vi "Begin.vi"() -> (0 "error out":errorcluster)   [LabVIEW 2013]
doc: "Called before other user functions, this VI is expected to open initial I/O refnums, load in file data, and do all program initialization. Notice that the <B>error out</B> terminal is simply used for data flow. Wiring it to other structures or subVIs ensures that this VI runs first."
uses:
  <vilib>/Rock Robotics/WPI/DriverStation/WPI_DriverStationRobotMode2.ctl
  <vilib>/Rock Robotics/WPI/Joystick/WPI_JoystickDeviceEnum.ctl
  <vilib>/Rock Robotics/SystemInterfaces/DIO/FPGA_DIOChannel.ctl
  <vilib>/Rock Robotics/SystemInterfaces/DIO/FPGA_DIORelayChannel.ctl
  <vilib>/Rock Robotics/SystemInterfaces/AI/FPGA_AIChannel.ctl
  <vilib>/Rock Robotics/SystemInterfaces/AI/FPGA_AIGyroChannel.ctl
  <vilib>/Rock Robotics/SystemInterfaces/Typedef/FPGA_TypedefAnalogModuleForGyro.ctl
  <vilib>/Rock Robotics/SystemInterfaces/Typedef/FPGA_TypedefDigitalModule.ctl
  <vilib>/Rock Robotics/SystemInterfaces/DIO/FPGA_DIOPWMChannel.ctl
  <vilib>/Rock Robotics/WPI/SafetyOutput/WPI_SafetyOutputConfigMenu.ctl
  <vilib>/Rock Robotics/WPI/Solenoid/WPI_SolenoidChannel.ctl
  <vilib>/Rock Robotics/WPI/Relay/WPI_RelayValue.ctl
  <vilib>/Rock Robotics/SystemInterfaces/Typedef/FPGA_TypedefAnalogModule.ctl
  <vilib>/Rock Robotics/WPI/Solenoid/WPI_SolenoidValue.ctl
  Robot Global Data.vi
  <vilib>/Rock Robotics/WPI/Counter/WPI_CounterDigitalInputToDigitalSource.vi
  <vilib>/Rock Robotics/WPI/RobotDrive/WPI_RobotDriveOpen2MotorWithTalon.vi
  <vilib>/Rock Robotics/WPI/MotorControl/WPI_MotorControlOpen Talon.vi
  <vilib>/Rock Robotics/WPI/Solenoid/WPI_SolenoidOpenSingle.vi
  <vilib>/Rock Robotics/WPI/Solenoid/WPI_SolenoidSetEnum.vi
  <vilib>/Rock Robotics/WPI/Compressor/WPI_CompressorGetSetRefNum.vi
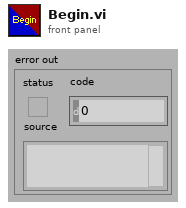
[diagram p1: front panel]
types:
  T1 = typedef "FPGA_DIOChannel.ctl" = enum8{"DIO 1", "DIO 2", "DIO 3", "DIO 4", "DIO 5", "DIO 6", "DIO 7", "DIO 8", "DIO 9", "DIO 10", "DIO 11", "DIO 12", "DIO 13", "DIO 14", "Invalid"}
  T2 = typedef "WPI_SolenoidChannel.ctl" = enum8{"Solenoid 1", "Solenoid 2", "Solenoid 3", "Solenoid 4", "Solenoid 5", "Solenoid 6", "Solenoid 7", "Solenoid 8", "Invalid"}
  T3 = typedef "WPI_SolenoidValue.ctl" = enum16{"Off", "On", "Forward", "Reverse"}
  T4 = typedef "FPGA_TypedefAnalogModule.ctl" = enum16{"Analog Module 1", "Analog Module 2"}
  T5 = typedef "FPGA_DIORelayChannel.ctl" = enum8{"Relay 1", "Relay 2", "Relay 3", "Relay 4", "Relay 5", "Relay 6", "Relay 7", "Relay 8", "Invalid"}
  T6 = typedef "WPI_RelayValue.ctl" = enum16{"Off", "On", "Forward", "Reverse"}
  T7 = typedef "FPGA_DIOPWMChannel.ctl" = enum8{"PWM 1", "PWM 2", "PWM 3", "PWM 4", "PWM 5", "PWM 6", "PWM 7", "PWM 8", "PWM 9", "PWM 10", "Invalid"}
  T8 = typedef "WPI_SafetyOutputConfigMenu.ctl" = enum16{"Enable", "Disable"}
  T9 = typedef "FPGA_TypedefDigitalModule.ctl" = enum16{"Digital Module 1", "Digital Module 2"}
  T10 = typedef "FPGA_TypedefAnalogModuleForGyro.ctl" = enum16{"Analog Module 1"}
  T11 = typedef "FPGA_AIGyroChannel.ctl" = enum8{"AI 1", "AI 2", "Invalid"}
  T12 = typedef "FPGA_AIChannel.ctl" = enum8{"AI 1", "AI 2", "AI 3", "AI 4", "AI 5", "AI 6", "AI 7", "AI 8", "Invalid"}
  T13 = typedef "WPI_JoystickDeviceEnum.ctl" = enum16{"USB 1", "USB 2", "USB 3", "USB 4", "Kinect 1", "Kinect 2"}
  T14 = typedef "WPI_DriverStationRobotMode2.ctl" = enum16{"Autonomous Disabled", "Autonomous Enabled", "Teleop Disabled", "Teleop Enabled", "Timeout", "Finish", "Test Disabled", "Test Enabled"}
  T15 = typedef "WPI_JoystickDevRef.ctl" = cluster{"Device":T13}
  T16 = typedef "WPI_SolenoidDevRef.ctl" = cluster{"DevStatus":errorcluster, "Solenoid Module":T17, "Forward Solenoid Channel":T2, "Reverse Solenoid Channel":T2}
  T17 = typedef "FPGA_TypedefSolenoidModule.ctl" = enum16{"Solenoid Module 1", "Solenoid Module 2"}
  T18 = typedef "WPI_CompressorDevRef.ctl" = cluster{"DevStatus":errorcluster, "DigitalInputDevRef":T19, "RelayDevRef":T20}
  T19 = typedef "WPI_DigitalInputDevRef.ctl" = cluster{"DevStatus":errorcluster, "DIO Channel":T1, "Digital Module":T9}
  T20 = typedef "WPI_RelayDevRef.ctl" = cluster{"DevStatus":errorcluster, "Relay Channel":T5, "Digital Module":T9, "Relay Direction":T21}
  T21 = typedef "WPI_RelayDirection.ctl" = enum16{"Both directions", "Forward only", "Reverse only"}
  T22 = typedef "FPGA_CounterEncoderSourceConvertionLVSourceType.ctl" = cluster{"DevStatus":errorcluster, "AnalogTriggerMode?":bool, "DigitalMode":cluster{"Digital Module":T9, "DIO Channel":T23}, "AnalogTriggerMode":cluster{"AnalogTriggerIndex":T24, "OutputType":T25}}
  T23 = typedef "FPGA_DIODigitalSourceChannel.ctl" = enum8{"DIO 1", "DIO 2", "DIO 3", "DIO 4", "DIO 5", "DIO 6", "DIO 7", "DIO 8", "DIO 9", "DIO 10", "DIO 11", "DIO 12", "DIO 13", "DIO 14", "Disabled"}
  T24 = typedef "FPGA_AnalogTriggerIndex.ctl" = enum8{"Trig 0", "Trig 1", "Trig 2", "Trig 3", "Trig 4", "Trig 5", "Trig 6", "Trig 7", "Invalid"}
  T25 = typedef "FPGA_AnalogTriggerOutType.ctl" = enum16{"InWindow", "TriggerState", "Rising", "Falling"}
  T26 = typedef "WPI_MotorControlDeviceRef.ctl" = cluster{"DeviceStatus":errorcluster, "Type":enum16{"PWM", "CAN"}, "PWM":cluster{"Digital Module":T9, "PWM Channel":T7, "DeadBand":T27}, "CAN":cluster{"Device Number":u8, "Control Mode":T28, "Semaphore":T29, "Max Vout":dbl}, "Invert":bool, "TransformRef":T30, "InvTransformRef":T30}
  T27 = typedef "WPI_PWMDeadband.ctl" = cluster{"Name":string, "maxPositivePwm":i32, "minPositivePwm":i32, "centerPwm":i32, "maxNegativePwm":i32, "minNegativePwm":i32, "angularRange":u16}
  T28 = typedef "WPI_CANJaguar_ControlMode.ctl" = enum8{"Percent VBus", "Current", "Speed", "Position", "Voltage"}
  T29 = typedef "Semaphore RefNum" = refnum<k1>
  T30 = typedef "WPI_PWMTransform_ConPane.ctl" = refnum<vi>
  T31 = typedef "WPI_RobotDriveDevRef.ctl" = cluster{"DevStatus":errorcluster, "Motors[]":T26[], "Square Inputs":bool, "Max Output":dbl, "Isochronous":bool}
  T32 = typedef "WPI_EncoderDevRef.ctl" = cluster{"DevStatus":errorcluster, "EncoderIndex":T33, "CounterIndex":T34, "DistancePerCount":dbl, "Decoding Type":T35}
  T33 = typedef "FPGA_EncoderIdx.ctl" = enum8{"Enc 0", "Enc 1", "Enc 2", "Enc 3", "Invalid"}
  T34 = typedef "FPGA_CounterCtrSystemIndex.ctl" = enum8{"Ctr 0", "Ctr 1", "Ctr 2", "Ctr 3", "Ctr 4", "Ctr 5", "Ctr 6", "Ctr 7", "Invalid"}
  T35 = typedef "WPI_EncoderType.ctl" = enum16{"1x", "2x", "4x"}
  T36 = typedef "WPI_AnalogChannelDevRef.ctl" = cluster{"DevStatus":errorcluster, "Analog Module":T4, "Analog Channel":T12}
  T37 = typedef "WPI_GyroDevRef.ctl" = cluster{"DevStatus":errorcluster, "Analog Module":T4, "Analog Channel":T12, "Offset":dbl, "Gain (VoltsPerDegree/Second)":dbl}
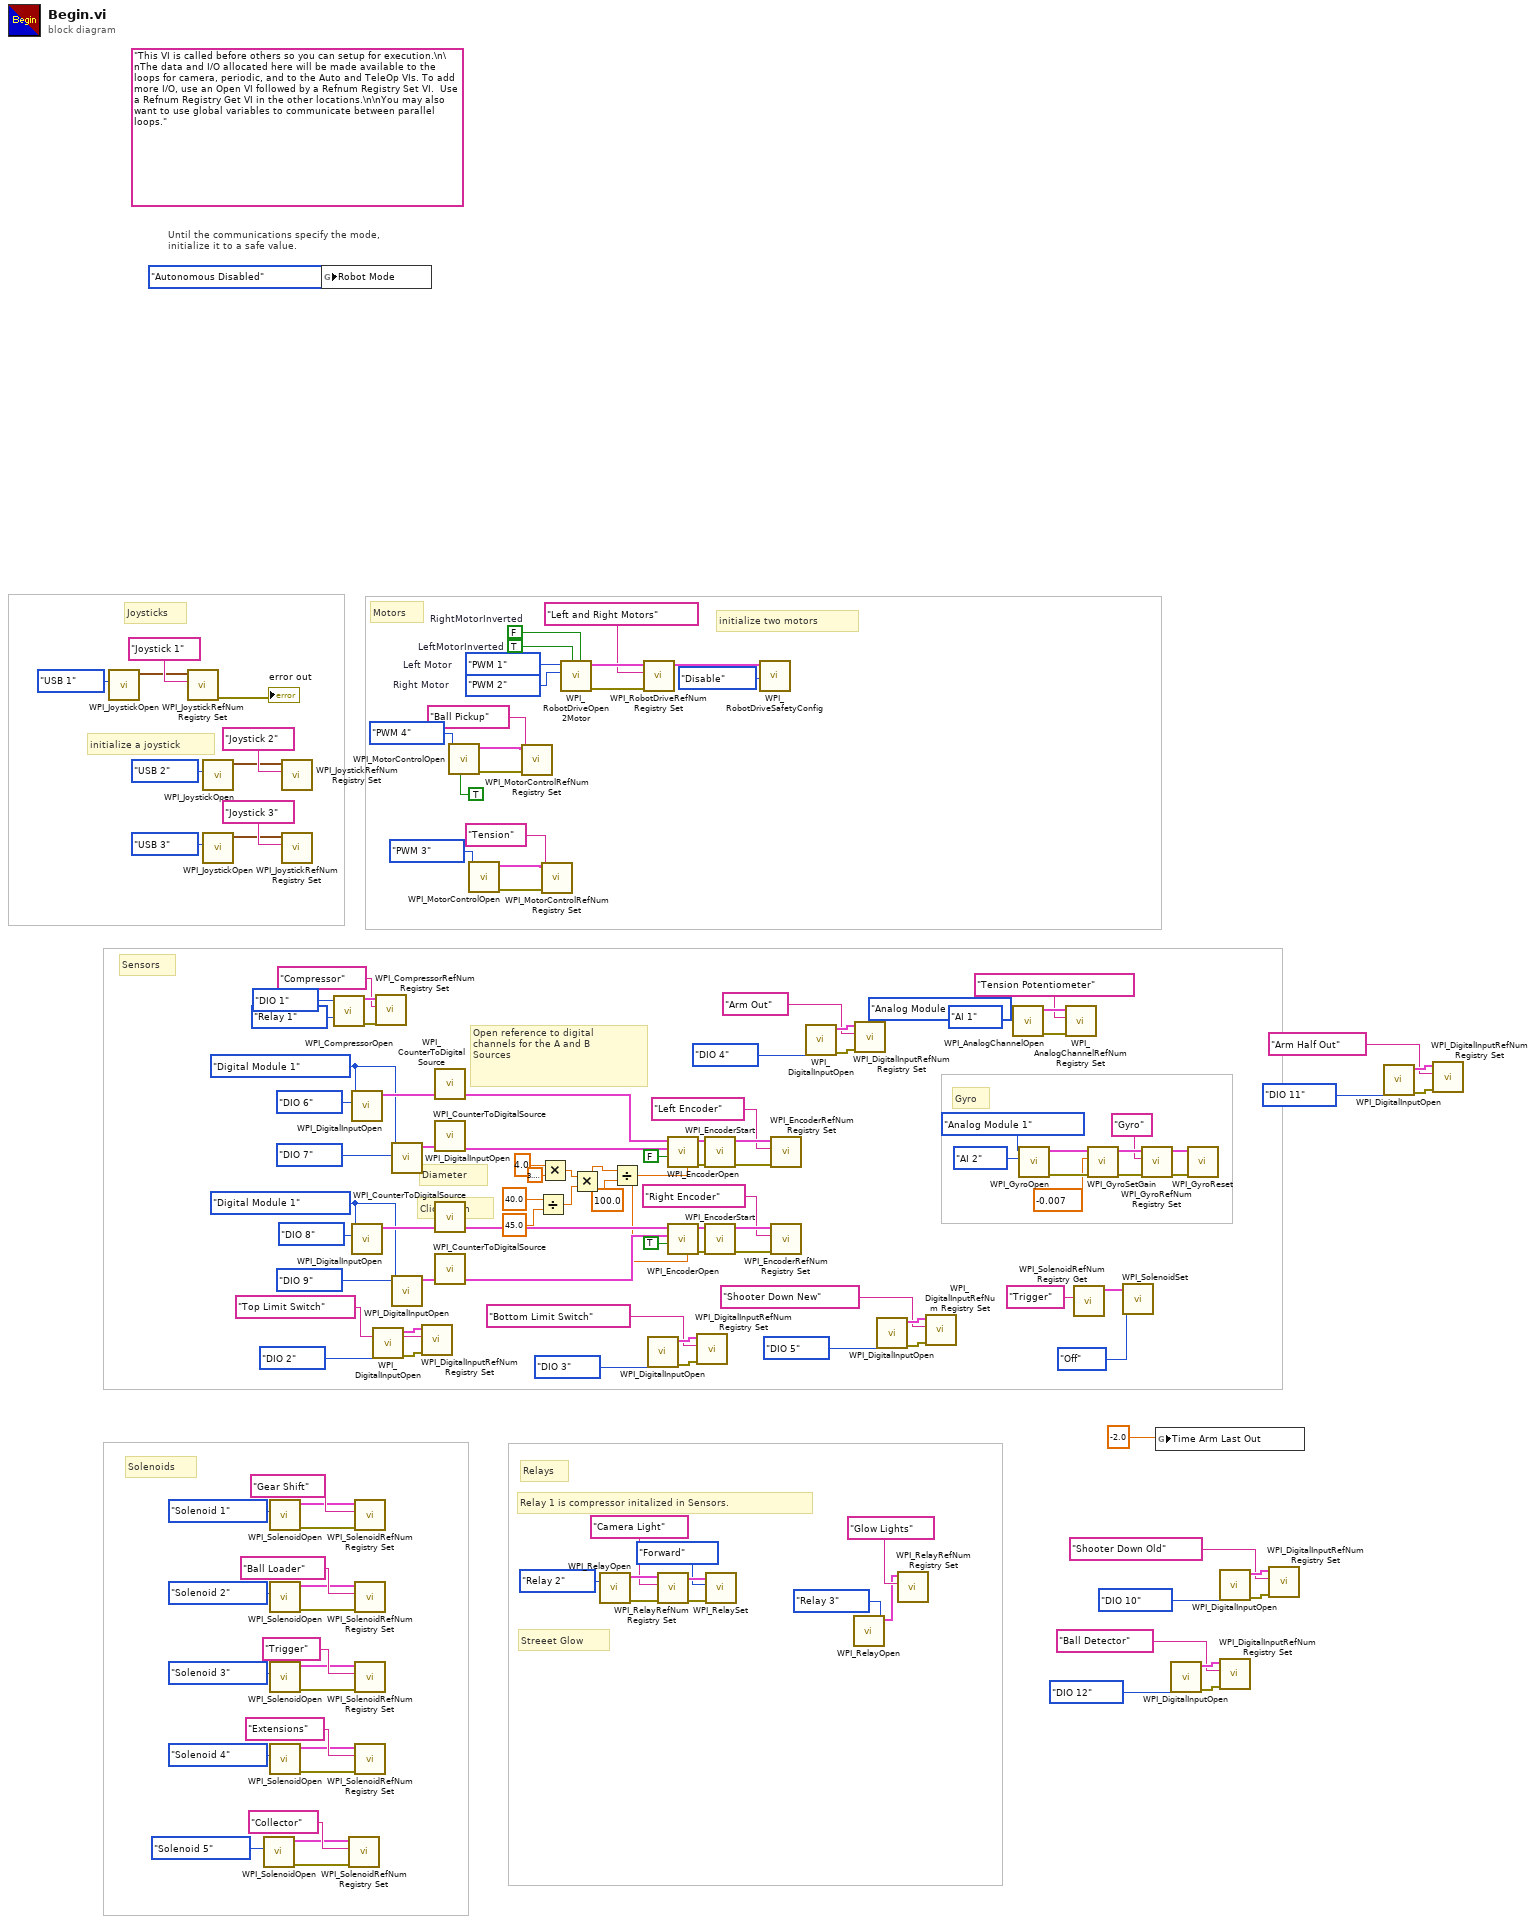
[diagram p0: block diagram]
diagram:
  w82 = FPGA_DIOPWMChannel."PWM 2"  # Right Motor
  w83 = FPGA_DIOPWMChannel."PWM 1"  # Left Motor
  w87 = TRUE  # LeftMotorInverted
  w88 = FALSE  # RightMotorInverted
  w96 = FPGA_TypedefDigitalModule."Digital Module 1" ("DIO Module 2")
  w103 = FPGA_TypedefDigitalModule."Digital Module 1" ("DIO Module")
  (unwired) "This VI is called before others so you can setup for execution.\n\nThe data and I/O allocated here will be made available to the loops for camera, periodic, and to the Auto and TeleOp VIs. To add more I/O, use an Open VI followed by a Refnum Registry Set VI.  Use a Refnum Registry Get VI in the other locations.\n\nYou may also want to use global variables to communicate between parallel loops."
  # "Streeet Glow"
  # "Relay 1 is compressor initalized in Sensors."
  # "Relays"
  # "Solenoids"
  # "Motors"
  # "initialize two motors"
  # "Clicks/inch"
  # "Diameter"
  # "Open reference to digital \nchannels for the A and B\nSources"
  # "Gyro"
  # "Sensors"
  # "Joysticks"
  # "initialize a joystick"
  # "Until the communications specify the mode,\ninitialize it to a safe value."
  n1 = call <vilib>:"WPI_JoystickOpen.vi"("JoystickDevice"=WPI_JoystickDeviceEnum."USB 1") -> ("JoystickDevRef"=w144:T15)  [unwired: 10 in]
  n2 = call <vilib>:"WPI_JoystickRefNum Registry Set.vi"("refnum name"="Joystick 1", "JoystickDevRef"=w144) -> ("error out"=→"error out":errorcluster)  [unwired: 8 in, 1 out]
  n3 = call <vilib>:"WPI_JoystickOpen.vi"("JoystickDevice"=WPI_JoystickDeviceEnum."USB 2") -> ("JoystickDevRef"=w140:T15)  [unwired: 10 in]
  n4 = call <vilib>:"WPI_JoystickOpen.vi"("JoystickDevice"=WPI_JoystickDeviceEnum."USB 3") -> ("JoystickDevRef"=w137:T15)  [unwired: 10 in]
  n5 = call-poly <vilib>:"WPI_SolenoidOpen.vi"("Solenoid Channel"=WPI_SolenoidChannel."Solenoid 5") -> ("error out"=w19:errorcluster, "SolenoidDevRef"=w20:T16)  [unwired: 9 in]
  n6 = call-poly <vilib>:"WPI_SolenoidOpen.vi"("Solenoid Channel"=WPI_SolenoidChannel."Solenoid 1") -> ("error out"=w55:errorcluster, "SolenoidDevRef"=w56:T16)  [unwired: 9 in]
  n7 = call-poly <vilib>:"WPI_SolenoidOpen.vi"("Solenoid Channel"=WPI_SolenoidChannel."Solenoid 2") -> ("error out"=w59:errorcluster, "SolenoidDevRef"=w60:T16)  [unwired: 9 in]
  n8 = call-poly <vilib>:"WPI_SolenoidOpen.vi"("Solenoid Channel"=WPI_SolenoidChannel."Solenoid 3") -> ("error out"=w63:errorcluster, "SolenoidDevRef"=w64:T16)  [unwired: 9 in]
  n9 = call-poly <vilib>:"WPI_SolenoidOpen.vi"("Solenoid Channel"=WPI_SolenoidChannel."Solenoid 4") -> ("error out"=w67:errorcluster, "SolenoidDevRef"=w68:T16)  [unwired: 9 in]
  n10 = call <vilib>:"WPI_JoystickRefNum Registry Set.vi"("refnum name"="Joystick 2", "JoystickDevRef"=w140) -> ()  [unwired: 8 in, 2 out]
  n11 = call <vilib>:"WPI_JoystickRefNum Registry Set.vi"("refnum name"="Joystick 3", "JoystickDevRef"=w137) -> ()  [unwired: 8 in, 2 out]
  n12 = global write "Robot Global Data.vi" "Robot Mode"(WPI_DriverStationRobotMode2."Autonomous Disabled" ("Robot Mode")) -> ()
  n13 = call <vilib>:"WPI_CompressorOpen.vi"("Pressure Switch DIO Channel"=FPGA_DIOChannel."DIO 1", "Relay Channel"=FPGA_DIORelayChannel."Relay 1") -> ("CompressorDevRef"=w134:T18, "error out"=w135:errorcluster)  [unwired: 12 in]
  n14 = call <vilib>:"WPI_SolenoidRefNum Registry Set.vi"("error in (no error)"=w19, "refnum name"="Collector", "SolenoidDevRef"=w20) -> ()  [unwired: 7 in, 2 out]
  n15 = call <vilib>:"WPI_DigitalInputOpen.vi"("DIO Channel"=FPGA_DIOChannel."DIO 6" ("A Channel"), "Digital Module (Module 1)"=w103) -> ("DigitalInputDevRef"=w106:T19)  [unwired: 1 in, 8 out]
  n16 = call <vilib>:"WPI_DigitalInputOpen.vi"("DIO Channel"=FPGA_DIOChannel."DIO 8" ("A Channel 2"), "Digital Module (Module 1)"=w96) -> ("DigitalInputDevRef"=w99:T19)  [unwired: 1 in, 8 out]
  n17 = call <vilib>:"WPI_SolenoidRefNum Registry Set.vi"("error in (no error)"=w55, "refnum name"="Gear Shift", "SolenoidDevRef"=w56) -> ()  [unwired: 7 in, 2 out]
  n18 = call <vilib>:"WPI_SolenoidRefNum Registry Set.vi"("error in (no error)"=w59, "refnum name"="Ball Loader", "SolenoidDevRef"=w60) -> ()  [unwired: 7 in, 2 out]
  n19 = call <vilib>:"WPI_SolenoidRefNum Registry Set.vi"("error in (no error)"=w63, "refnum name"="Trigger", "SolenoidDevRef"=w64) -> ()  [unwired: 7 in, 2 out]
  n20 = call <vilib>:"WPI_SolenoidRefNum Registry Set.vi"("error in (no error)"=w67, "refnum name"="Extensions", "SolenoidDevRef"=w68) -> ()  [unwired: 7 in, 2 out]
  n21 = call <vilib>:"WPI_DigitalInputOpen.vi"("DIO Channel"=FPGA_DIOChannel."DIO 2") -> ("error out"=w43:errorcluster, "DigitalInputDevRef"=w42:T19)  [unwired: 9 in]
  n22 = call <vilib>:"WPI_CompressorRefNum Registry Set.vi"("error in (no error)"=w135, "refnum name"="Compressor", "CompressorDevRef"=w134) -> ()  [unwired: 7 in, 2 out]
  n23 = call <vilib>:"WPI_DigitalInputOpen.vi"("DIO Channel"=FPGA_DIOChannel."DIO 7" ("B Channel"), "Digital Module (Module 1)"=w103) -> ("DigitalInputDevRef"=w107:T19)  [unwired: 1 in, 8 out]
  n24 = call <vilib>:"WPI_DigitalInputOpen.vi"("DIO Channel"=FPGA_DIOChannel."DIO 9" ("B Channel 2"), "Digital Module (Module 1)"=w96) -> ("DigitalInputDevRef"=w100:T19)  [unwired: 1 in, 8 out]
  n25 = call <vilib>:"WPI_DigitalInputRefNum Registry Set.vi"("error in (no error)"=w43, "refnum name"="Top Limit Switch", "DigitalInputDevRef"=w42) -> ()  [unwired: 7 in, 2 out]
  n26 = call-poly <vilib>:"WPI_CounterToDigitalSource.vi"("DigitalInputDevRef"=w106) -> ("Digital Source"=w102:T22)  [unwired: 6 out]
  n27 = call-poly <vilib>:"WPI_CounterToDigitalSource.vi"("DigitalInputDevRef"=w107) -> ("Digital Source"=w101:T22)  [unwired: 6 out]
  n28 = call-poly <vilib>:"WPI_CounterToDigitalSource.vi"("DigitalInputDevRef"=w99) -> ("Digital Source"=w95:T22)  [unwired: 6 out]
  n29 = call-poly <vilib>:"WPI_CounterToDigitalSource.vi"("DigitalInputDevRef"=w100) -> ("Digital Source"=w94:T22)  [unwired: 6 out]
  n30 = call-poly <vilib>:"WPI_MotorControlOpen.vi"("Invert"=TRUE, "PWM Channel"=FPGA_DIOPWMChannel."PWM 4") -> ("error out"=w72:errorcluster, "MotorControlDeviceRef"=w75:T26)  [unwired: 8 in]
  n31 = call-poly <vilib>:"WPI_MotorControlOpen.vi"("PWM Channel"=FPGA_DIOPWMChannel."PWM 3") -> ("error out"=w76:errorcluster, "MotorControlDeviceRef"=w79:T26)  [unwired: 9 in]
  n32 = call <vilib>:"WPI_MotorControlRefNum Registry Set.vi"("error in (no error)"=w72, "refnum name"="Ball Pickup", "MotorControlDevRef"=w75) -> ()  [unwired: 7 in, 2 out]
  n33 = Divide(x=40.0, y=45.0) -> (x/y=w13:dbl)
  n34 = Multiply(x=4.0, y=3.141592653589793) -> (x*y=w14:dbl)
  n35 = call <vilib>:"WPI_MotorControlRefNum Registry Set.vi"("error in (no error)"=w76, "refnum name"="Tension", "MotorControlDevRef"=w79) -> ()  [unwired: 7 in, 2 out]
  n36 = call-poly <vilib>:"WPI_RobotDriveOpen2Motor.vi"("Right Motor Inverted"=w88, "Left Motor Inverted"=w87, "Right Motor"=w82, "Left Motor"=w83) -> ("error out"=w84:errorcluster, "RobotDriveDevRef"=w86:T31)  [unwired: 1 in, 5 out]
  n37 = Multiply(x=w14, y=w13) -> (x*y=w15:dbl)
  n38 = call <vilib>:"WPI_RelayOpen.vi"("Relay Channel"=FPGA_DIORelayChannel."Relay 2") -> ("error out"=w54:errorcluster, "RelayDevRef"=w53:T20)  [unwired: 9 in]
  n39 = Divide(x=w15, y=100.0) -> (x/y=w91:dbl)
  n40 = call <vilib>:"WPI_RobotDriveRefNum Registry Set.vi"("error in (no error)"=w84, "refnum name"="Left and Right Motors", "RobotDriveDevRef"=w86) -> ("RobotDriveDevRef"=w81:T31)  [unwired: 8 out]
  n41 = call <vilib>:"WPI_DigitalInputOpen.vi"("DIO Channel"=FPGA_DIOChannel."DIO 3") -> ("error out"=w39:errorcluster, "DigitalInputDevRef"=w38:T19)  [unwired: 9 in]
  n42 = call <vilib>:"WPI_RelayRefNum Registry Set.vi"("error in (no error)"=w54, "refnum name"="Camera Light", "RelayDevRef"=w53) -> ("error out"=w49:errorcluster, "RelayDevRef"=w50:T20)  [unwired: 7 in]
  n43 = call <vilib>:"WPI_EncoderOpen.vi"("DistancePerCount"=w91, "Invert Direction (False)"=FALSE, "BSource"=w101, "ASource"=w102) -> ("error out"=w116:errorcluster, "EncoderDevRef"=w115:T32)  [unwired: 6 in]
  n44 = call <vilib>:"WPI_EncoderOpen.vi"("DistancePerCount"=w91, "Invert Direction (False)"=TRUE, "BSource"=w94, "ASource"=w95) -> ("error out"=w112:errorcluster, "EncoderDevRef"=w111:T32)  [unwired: 6 in]
  n45 = call <vilib>:"WPI_DigitalInputRefNum Registry Set.vi"("error in (no error)"=w39, "refnum name"="Bottom Limit Switch", "DigitalInputDevRef"=w38) -> ()  [unwired: 7 in, 2 out]
  n46 = call <vilib>:"WPI_EncoderStart.vi"("error in (no error)"=w116, "EncoderDevRef"=w115) -> ("error out"=w114:errorcluster, "EncoderDevRef"=w113:T32)  [unwired: 8 in]
  n47 = call <vilib>:"WPI_EncoderStart.vi"("error in (no error)"=w112, "EncoderDevRef"=w111) -> ("error out"=w110:errorcluster, "EncoderDevRef"=w109:T32)  [unwired: 8 in]
  n48 = call <vilib>:"WPI_RelaySet.vi"("error in (no error)"=w49, "RelayValue"=WPI_RelayValue."Forward", "RelayDevRef"=w50) -> ()  [unwired: 7 in, 2 out]
  n49 = call <vilib>:"WPI_RobotDriveSafetyConfig.vi"("mode"=WPI_SafetyOutputConfigMenu."Disable", "RobotDriveDevRef"=w81) -> ()  [unwired: 8 in, 2 out]
  n50 = call <vilib>:"WPI_EncoderRefNum Registry Set.vi"("error in (no error)"=w114, "refnum name"="Left Encoder", "EncoderDevRef"=w113) -> ()  [unwired: 7 in, 2 out]
  n51 = call <vilib>:"WPI_EncoderRefNum Registry Set.vi"("error in (no error)"=w110, "refnum name"="Right Encoder", "EncoderDevRef"=w109) -> ()  [unwired: 7 in, 2 out]
  n52 = call <vilib>:"WPI_DigitalInputOpen.vi"("DIO Channel"=FPGA_DIOChannel."DIO 4") -> ("error out"=w34:errorcluster, "DigitalInputDevRef"=w33:T19)  [unwired: 9 in]
  n53 = call <vilib>:"WPI_RelayOpen.vi"("Relay Channel"=FPGA_DIORelayChannel."Relay 3") -> ("RelayDevRef"=w45:T20)  [unwired: 9 in, 1 out]
  n54 = call <vilib>:"WPI_DigitalInputRefNum Registry Set.vi"("error in (no error)"=w34, "refnum name"="Arm Out", "DigitalInputDevRef"=w33) -> ()  [unwired: 7 in, 2 out]
  n55 = call <vilib>:"WPI_DigitalInputOpen.vi"("DIO Channel"=FPGA_DIOChannel."DIO 5") -> ("error out"=w30:errorcluster, "DigitalInputDevRef"=w29:T19)  [unwired: 9 in]
  n56 = call <vilib>:"WPI_RelayRefNum Registry Set.vi"("refnum name"="Glow Lights", "RelayDevRef"=w45) -> ()  [unwired: 8 in, 2 out]
  n57 = call <vilib>:"WPI_DigitalInputRefNum Registry Set.vi"("error in (no error)"=w30, "refnum name"="Shooter Down New", "DigitalInputDevRef"=w29) -> ()  [unwired: 7 in, 2 out]
  n58 = call <vilib>:"WPI_AnalogChannelOpen.vi"("Analog Channel"=FPGA_AIChannel."AI 1", "Analog Module (Module 1)"=FPGA_TypedefAnalogModule."Analog Module 1") -> ("error out"=w130:errorcluster, "AIDeviceRef"=w129:T36)  [unwired: 8 in]
  n59 = call <vilib>:"WPI_GyroOpen.vi"("Analog Channel"=FPGA_AIGyroChannel."AI 2", "Analog Module (Module 1)"=FPGA_TypedefAnalogModuleForGyro."Analog Module 1") -> ("error out"=w124:errorcluster, "GyroDevRef"=w123:T37)  [unwired: 7 in, 1 out]
  n60 = call <vilib>:"WPI_AnalogChannelRefNum Registry Set.vi"("error in (no error)"=w130, "refnum name"="Tension Potentiometer", "AIDeviceRef"=w129) -> ()  [unwired: 7 in, 2 out]
  n61 = call <vilib>:"WPI_SolenoidRefNum Registry Get.vi"("refnum name"="Trigger") -> ("SolenoidDevRef"=w25:T16)  [unwired: 9 in, 1 out]
  n62 = call <vilib>:"WPI_GyroSetGain.vi"("error in (no error)"=w124, "Gain (VoltsPerDegree/Second)"=-0.007, "GyroDevRef"=w123) -> ("error out"=w121:errorcluster, "GyroDevRef"=w120:T37)  [unwired: 7 in]
  n63 = call-poly <vilib>:"WPI_SolenoidSet.vi"("Value"=WPI_SolenoidValue."Off", "SolenoidDevRef"=w25) -> ()  [unwired: 8 in, 2 out]
  n64 = call <vilib>:"WPI_GyroRefNum Registry Set.vi"("error in (no error)"=w121, "refnum name"="Gyro", "GyroDevRef"=w120) -> ("error out"=w118:errorcluster, "GyroDevRef"=w117:T37)  [unwired: 7 in]
  n65 = global write "Robot Global Data.vi" "Time Arm Last Out"(-2.0 ("Time Arm Last Out")) -> ()
  n66 = call <vilib>:"WPI_DigitalInputOpen.vi"("DIO Channel"=FPGA_DIOChannel."DIO 12") -> ("error out"=w4:errorcluster, "DigitalInputDevRef"=w3:T19)  [unwired: 9 in]
  n67 = call <vilib>:"WPI_GyroReset.vi"("error in (no error)"=w118, "GyroDevRef"=w117) -> ()  [unwired: 8 in, 2 out]
  n68 = call <vilib>:"WPI_DigitalInputOpen.vi"("DIO Channel"=FPGA_DIOChannel."DIO 10") -> ("error out"=w8:errorcluster, "DigitalInputDevRef"=w7:T19)  [unwired: 9 in]
  n69 = call <vilib>:"WPI_DigitalInputRefNum Registry Set.vi"("error in (no error)"=w4, "refnum name"="Ball Detector", "DigitalInputDevRef"=w3) -> ()  [unwired: 7 in, 2 out]
  n70 = call <vilib>:"WPI_DigitalInputRefNum Registry Set.vi"("error in (no error)"=w8, "refnum name"="Shooter Down Old", "DigitalInputDevRef"=w7) -> ()  [unwired: 7 in, 2 out]
  n71 = call <vilib>:"WPI_DigitalInputOpen.vi"("DIO Channel"=FPGA_DIOChannel."DIO 11") -> ("error out"=w12:errorcluster, "DigitalInputDevRef"=w11:T19)  [unwired: 9 in]
  n72 = call <vilib>:"WPI_DigitalInputRefNum Registry Set.vi"("error in (no error)"=w12, "refnum name"="Arm Half Out", "DigitalInputDevRef"=w11) -> ()  [unwired: 7 in, 2 out]
